vi "Create Message Data Clusters (complex).vi"(8 "error in (no error)":errorcluster, 9 "generate serialization helpers":bool, 10 "message metadata":T1, 11 "library in":refnum<vi>) -> (0 "error out":errorcluster, 3 "library out":refnum<vi>)   [LabVIEW 2019, in "gRPC Template Creation Utility.lvlib"]
uses:
  gRPC Template Creation Utility.lvlib
  TypeDefs/Message Metadata (Scripting).ctl
  TypeDefs/Message Element Type.ctl
  TypeDefs/Message Element Metadata (Scripting).ctl
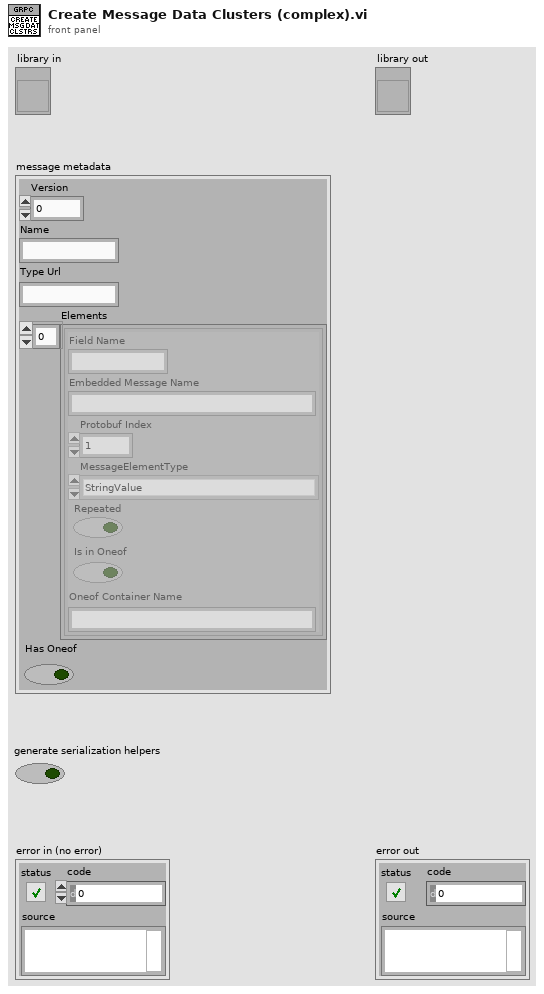
[diagram p1: front panel]
types:
  T1 = typedef "gRPC Template Creation Utility.lvlib/Message Metadata (Scripting).ctl" = cluster{"Version":i32, "Name":string, "Type Url":string, "Elements":T2[], "Has Oneof":bool}
  T2 = typedef "gRPC Template Creation Utility.lvlib/Message Element Metadata (Scripting).ctl" = cluster{"Field Name":string, "Embedded Message Name":string, "Protobuf Index":i32, "MessageElementType":T3, "Repeated":bool, "Is in Oneof":bool, "Oneof Container Name":string}
  T3 = typedef "gRPC Template Creation Utility.lvlib/Message Element Type.ctl" = enum32{"Int32Value", "FloatValue", "DoubleValue", "BoolValue", "StringValue", "MessageValue", "Int64Value", "UInt32Value", "UInt64Value", "EnumValue", "Bytes", "Fixed64", "Fixed32", "SFixed64", "SFixed32", "SInt64", "SInt32"}
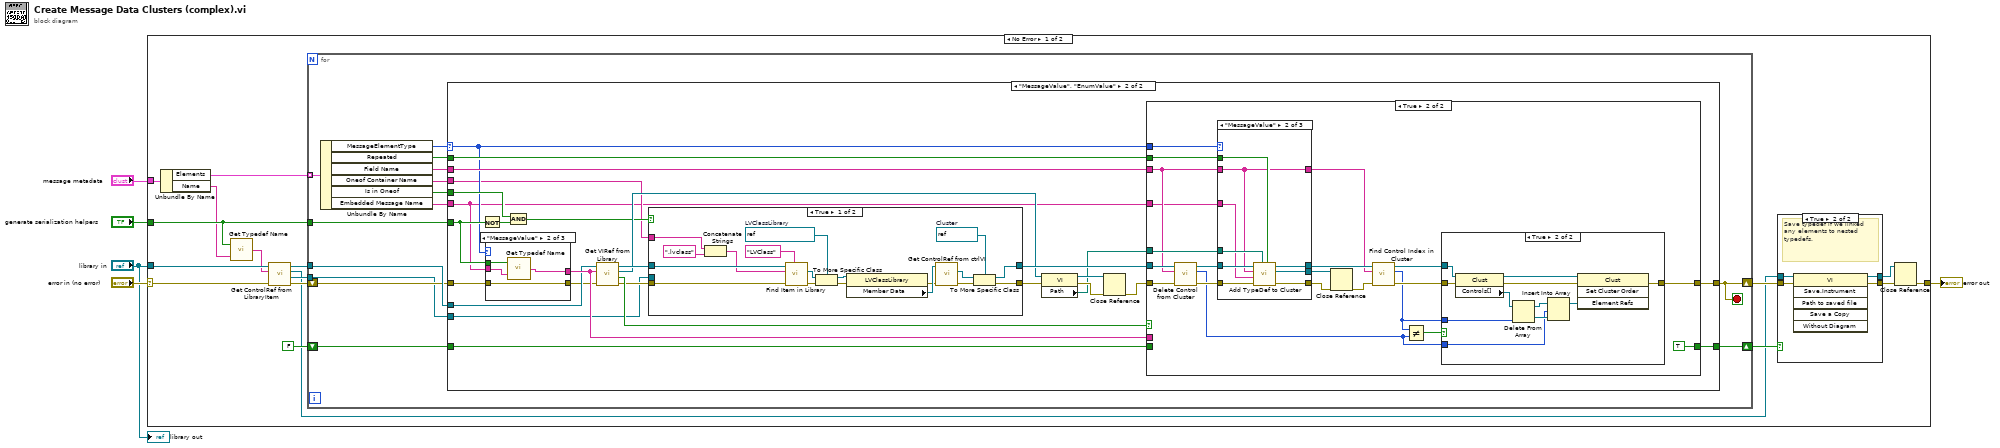
[diagram p0: block diagram]
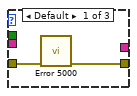
[diagram p4: hidden frame]
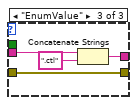
[diagram p5: hidden frame]
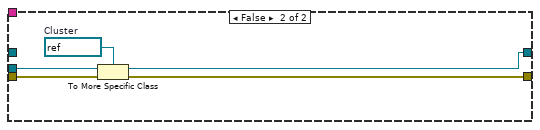
[diagram p6: hidden frame]
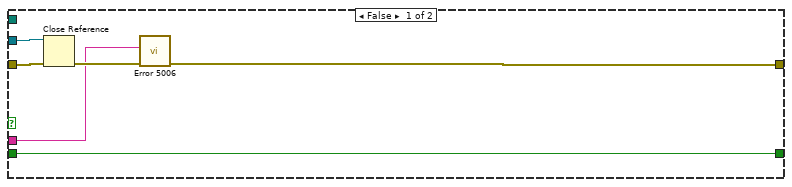
[diagram p7: hidden frame]
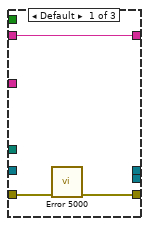
[diagram p8: hidden frame]
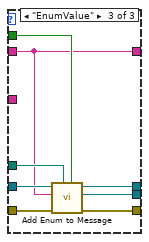
[diagram p9: hidden frame]
diagram:
  n1 = case shown="No Error" "error in (no error)" {
    selector: "error in (no error)" -> [w18 w164]
    tunnel: "message metadata" -> [w22 _]
    tunnel: "library in" -> [w16 _]
    tunnel: [w8 w164] -> w4
    tunnel: "generate serialization helpers" -> [w20 _]
    frame No Error {
      n2 = Unbundle By Name(w22) -> ("Elements"=w21:T2[], "Name"=w19:string)
      n3 = call "Get Typedef Name.vi"("embedded message name"=w19, "generate serialization helpers"=w20) -> ("typedef name"=w14:string)
      n4 = call "Get ControlRef from LibraryItem.vi"("error in (no error)"=w18, "Control Name"=w14, "Library item in"=w16) -> ("error out"=w17:errorcluster, "Control ref out"=w13:refnum<vi>, "VI ref out"=w6:refnum<vi>, "Library item out"=w15:refnum<vi>)  [unwired: 4 in, 1 out]
      n5 = for {
        tunnel: w21 -> [w41] mode=indexing
        shift-right: [w39] -> w10
        shift-left: w17 -> [w40]
        tunnel: w20 -> [w38]
        tunnel: w15 -> [w42]
        tunnel: w13 -> [w31]
        shift-right: [w29] -> w11
        shift-left: FALSE ("generate serialization helpers") -> [w30]
        stop <- w39 stop-if-true
        n6 = Unbundle By Name(w41) -> ("MessageElementType"=w34:T3, "Repeated"=w37:bool, "Field Name"=w36:string, "Oneof Container Name"=w35:string, "Is in Oneof"=w32:bool, "Embedded Message Name"=w33:string)
        n7 = case shown="\"MessageValue\", \"EnumValue\"" w34 {
          selector: w34 -> [_ w52]
          tunnel: w42 -> [_ w49]
          tunnel: w40 -> [w44 w53]
          tunnel: [w44 w59] -> w39
          tunnel: w38 -> [_ w66]
          tunnel: w37 -> [_ w56]
          tunnel: w36 -> [_ w55]
          tunnel: w32 -> [_ w54]
          tunnel: w35 -> [_ w51]
          tunnel: w33 -> [_ w50]
          tunnel: w31 -> [_ w47]
          tunnel: w30 -> [w43 w46]
          tunnel: [w43 w45] -> w29
          frame Default {
          }
          frame "MessageValue", "EnumValue" {
            n8 = Not(x=w66) -> (.not. x?=w65:bool)
            n9 = case shown="\"MessageValue\"" w52 {
              tunnel: [_ w77 w79] -> w71
              tunnel: w66 -> [_ w76 _]
              tunnel: w50 -> [_ w75 w80]
              tunnel: w53 -> [w73 w74 w78]
              tunnel: [w72 w74 w78] -> w48
              frame Default {
                n10 = call "Error 5000.vi"("error in (no error)"=w73) -> ("error out"=w72:errorcluster)  [unwired: 10 in]
              }
              frame "MessageValue" {
                n11 = call "Get Typedef Name.vi"("embedded message name"=w75, "generate serialization helpers"=w76) -> ("typedef name"=w77:string)
              }
              frame "EnumValue" {
                n12 = Concatenate Strings(w80, ".ctl" ("string")) -> (w79:string)
              }
            }
            n13 = And(x=w54, y=w65) -> (x .and. y?=w57:bool)
            n14 = call "Get VIRef from Library.vi"("error in (no error)"=w48, "item name"=w71, "library in"=w49) -> ("error out"=w68:errorcluster, "found"=w69:bool, "vi"=w64:refnum<vi>, "library out"=w67:refnum<vi>)  [unwired: 5 in]
            n15 = case shown="True" w57 {
              tunnel: w47 -> [_ w104]
              tunnel: [w90 w102] -> w70
              tunnel: w68 -> [w97 w101]
              tunnel: [w83 w100] -> w60
              tunnel: w67 -> [w99 _]
              tunnel: w51 -> [w89 _]
              frame True {
                w91 = refnum<vi> refnum  # Cluster
                w96 = refnum<vi> refnum  # LVClassLibrary
                n16 = Concatenate Strings(w89, ".lvclass" ("string")) -> (w87:string)
                n17 = call "Find Item in Library.vi"("Item Type"="LVClass", "error in (no error)"=w97, "Item Name"=w87, "Library item in"=w99) -> ("error out"=w95:errorcluster, "Project Item (Library Item)"=w94:refnum<vi>)  [unwired: 4 in, 2 out]
                n18 = To More Specific Class(target class=w96, reference=w94, error in=w95) -> (specific class reference=w93:refnum<vi>, error out=w92:errorcluster)
                n19 = property class="LVClassLibrary"(reference=w93, error in=w92) -> (error out=w84:errorcluster, "Member Data"=w86:refnum<vi>)  [unwired: 1 out]
                n20 = call "Get ControlRef from ctrlVI.vi"("error in (no error)"=w84, "VI ref in"=w86) -> ("error out"=w82:errorcluster, "Control ref out"=w85:refnum<vi>)  [unwired: 7 in, 1 out]
                n21 = To More Specific Class(target class=w91, reference=w85, error in=w82) -> (specific class reference=w90:refnum<vi>, error out=w83:errorcluster)
              }
              frame False {
                w103 = refnum<vi> refnum  # Cluster
                n22 = To More Specific Class(target class=w103, reference=w104, error in=w101) -> (specific class reference=w102:refnum<vi>, error out=w100:errorcluster)
              }
            }
            n23 = property class="VI"(reference=w64, error in=w60) -> (reference out=w62:refnum<vi>, error out=w63:errorcluster, "Path"=w58:path)
            n24 = Close Reference(reference=w62, error in (no error)=w63) -> (error out=w61:errorcluster)
            n25 = case shown="True" w69 {
              tunnel: w70 -> [w110 w131]
              tunnel: [w107 w111] -> w59
              tunnel: w61 -> [w109 w126]
              tunnel: w55 -> [_ w115]
              tunnel: w56 -> [_ w118]
              tunnel: w71 -> [w106 _]
              tunnel: w58 -> [_ w117]
              tunnel: w52 -> [_ w116]
              tunnel: w50 -> [_ w113]
              tunnel: w46 -> [w105 _]
              tunnel: [w105 TRUE ("generate serialization helpers")] -> w45
              frame False {
                n26 = Close Reference(reference=w110, error in (no error)=w109) -> (error out=w108:errorcluster)
                n27 = call "Error 5006.vi"("error in (no error)"=w108, "Embedded Message Name"=w106) -> ("error out"=w107:errorcluster)  [unwired: 9 in]
              }
              frame True {
                n28 = call "Delete Control from Cluster.vi"("error in (no error)"=w126, "Control Name in"=w115, "Cluster ref in"=w131) -> ("error out"=w125:errorcluster, "Deleted Index"=w119:i32, "Cluster ref out"=w124:refnum<vi>)  [unwired: 6 in]
                n29 = case shown="\"MessageValue\"" w116 {
                  tunnel: w125 -> [w134 w143 w151]
                  tunnel: w124 -> [_ w142 w147]
                  tunnel: [_ w141 w149] -> w123
                  tunnel: [_ w140 w148] -> w122
                  tunnel: [w133 w139 w150] -> w121
                  tunnel: w118 -> [_ w138 w146]
                  tunnel: w117 -> [_ w137 w145]
                  tunnel: w115 -> [w132 w136 w144]
                  tunnel: [w132 w136 w144] -> w114
                  tunnel: w113 -> [_ w135 _]
                  frame Default {
                    n30 = call "Error 5000.vi"("error in (no error)"=w134) -> ("error out"=w133:errorcluster)  [unwired: 10 in]
                  }
                  frame "MessageValue" {
                    n31 = call "Add TypeDef to Cluster.vi"("isArray (F)"=w138, "TypeDef path"=w137, "error in (no error)"=w143, "field message name"=w135, "Field Name"=w136, "Owning cluster ref in"=w142) -> ("error out"=w139:errorcluster, "Control ref out"=w140:refnum<vi>, "Owning cluster ref out"=w141:refnum<vi>)  [unwired: 3 in]
                  }
                  frame "EnumValue" {
                    n32 = call "Add Enum to Message.vi"("isArray (F)"=w146, "TypeDef path"=w145, "error in (no error)"=w151, "Field Name"=w144, "Owning cluster ref in"=w147) -> ("error out"=w150:errorcluster, "Control ref out"=w148:refnum<vi>, "Owning cluster ref out"=w149:refnum<vi>)  [unwired: 4 in]
                  }
                }
                n33 = Close Reference(reference=w122, error in (no error)=w121) -> (error out=w120:errorcluster)
                n34 = call "Find Control Index in Cluster.vi"("error in (no error)"=w120, "Control Name"=w114, "Cluster ref in"=w123) -> ("error out"=w128:errorcluster, "Control Index"=w127:i32, "Cluster ref out"=w129:refnum<vi>)  [unwired: 6 in]
                n35 = Not Equal?(x=w127, y=w119) -> (x != y?=w130:bool)
                n36 = case shown="True" w130 {
                  tunnel: w129 -> [_ w163]
                  tunnel: w128 -> [w152 w162]
                  tunnel: w127 -> [_ w161]
                  tunnel: w119 -> [_ w158]
                  tunnel: [w152 w153] -> w111
                  frame False {
                  }
                  frame True {
                    n37 = property class="Clust"(reference=w163, error in=w162) -> (reference out=w157:refnum<vi>, error out=w154:errorcluster, "Controls[]"=w155:refnum<vi>[])
                    n38 = Delete From Array(array=w155, index=w161) -> (deleted portion=w159:refnum<vi>, array with subset deleted=w160:refnum<vi>[])  [unwired: 1 in]
                    n39 = Insert Into Array(array=w160, index=w158, new element=w159) -> (w156:refnum<vi>[])
                    n40 = invoke class="Clust" method="Set Cluster Order"(reference=w157, error in=w154, "Element Refs"=w156) -> (error out=w153:errorcluster)  [unwired: 1 in, 3 out]
                  }
                }
              }
            }
          }
        }
      }
      n41 = case shown="True" w11 {
        tunnel: w10 -> [w24 w28]
        tunnel: [w24 w27] -> w9
        tunnel: [w23 w26] -> w7
        tunnel: w6 -> [w23 w25]
        frame False {
        }
        frame True {
          # "Save typedef if we linked any elements to nested typedefs."
          n42 = invoke class="VI" method="Save.Instrument"(reference=w25, error in=w28) -> (reference out=w26:refnum<vi>, error out=w27:errorcluster)  [unwired: 4 in, 4 out]
        }
      }
      n43 = Close Reference(reference=w7, error in (no error)=w9) -> (error out=w8:errorcluster)
    }
    frame Error {
    }
  }
  "error out" <- w4
  "library out" <- "library in"
